vi "Joystick.vi"(1 "Joystick Refnum In":string="Joystick 1") -> (0 "Speed Out":dbl)   [LabVIEW 2012]
uses:
  Robot Global Data.vi
  <vilib>/Rock Robotics/WPI/Joystick/WPI_JoystickGetSetRefNum.vi
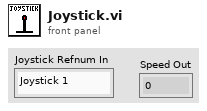
[diagram p1: front panel]
types:
  T1 = typedef "WPI_JoystickDevRef.ctl" = cluster{"Device":T2}
  T2 = typedef "WPI_JoystickDeviceEnum.ctl" = enum16{"USB 1", "USB 2", "USB 3", "USB 4", "Kinect 1", "Kinect 2"}
  T3 = cluster{"axis 1 (x)":dbl, "axis 2 (y)":dbl, "axis 3 (throttle)":dbl, "axis 4":dbl, "axis 5":dbl, "axis 6":dbl}
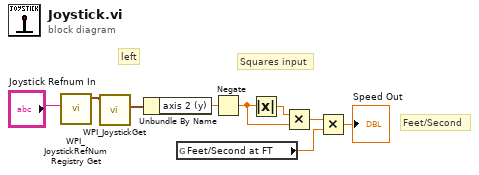
[diagram p0: block diagram]
diagram:
  # "Feet/Second"
  # "Squares input"
  # "left"
  n1 = call <vilib>:"WPI_JoystickRefNum Registry Get.vi"("refnum name"="Joystick Refnum In") -> ("JoystickDevRef"=w8:T1)  [unwired: 9 in, 1 out]
  n2 = call <vilib>:"WPI_JoystickGet.vi"("JoystickDevRef"=w8) -> ("Axes"=w7:T3)  [unwired: 4 in, 2 out]
  n3 = Unbundle By Name(w7) -> ("axis 2 (y)"=w4:dbl)
  n4 = global read "Robot Global Data.vi" "Feet/Second at FT"() -> (w5:dbl)
  n5 = Negate(x=w4) -> (-x=w2:dbl)
  n6 = Absolute Value(x=w2) -> (abs(x)=w3:dbl)
  n7 = Multiply(x=w3, y=w2) -> (x*y=w1:dbl)
  n8 = Multiply(x=w1, y=w5) -> (x*y=→"Speed Out":dbl)
